vi "cometPlot.vi"(7 "sortMethod":string, 11 "sortedCoords":sgl[][](array[numeric])) -> (3 "3D Comet":refnum<class "3D Plot Datatype.lvclass">[](xcontrol))   [LabVIEW 2021]
uses:
  <vilib>/Math Plots/3D Math Plots/3D Comet/3D Comet XCtrl/3D Comet.xctl
  <vilib>/Math Plots/3D Math Plots/3D Comet/3D Comet Datatype/Public/Plot Helper (Vector).vi
  <vilib>/Math Plots/3D Math Plots/3D Comet/3D Comet Datatype/3D Comet Datatype.lvclass
panel:
  # "(Right-click and \"Render Window\" to launch resizeable window)"
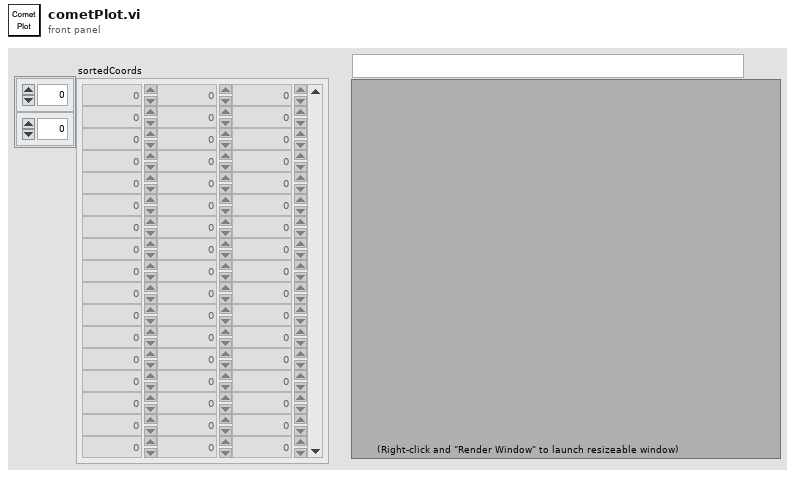
[diagram p1: front panel]
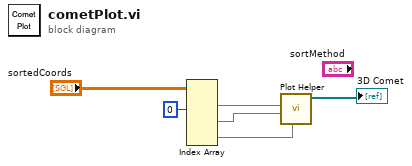
[diagram p0: block diagram]
diagram:
  n1 = Index Array(array="sortedCoords", index (col) #1=0 ("disabled index (col)")) -> (element #1=w3:sgl[], element #2=w4:sgl[], element #3=w5:sgl[])  [unwired: 5 in]
  n2 = call-poly <vilib>:"Plot Helper.vi"("z vector"=w5, "y vector"=w4, "x vector"=w3) -> ("3D Plot lvclass Array out"=→"3D Comet":refnum<class "3D Plot Datatype.lvclass">[])  [unwired: 3 in, 5 out]
